vi "Remove Headers from XML.vi"(8 "error in (no error)":errorcluster, 10 "XML (with headers)":string) -> (0 "error out":errorcluster, 2 "XML (without headers)":string)   [LabVIEW 2013]
panel:
  # "Copyright © 2007 James Kring, Inc. All rights reserved.\n\nAuthor: Jim Kring <jim.kring@jameskring.com>\n\nThis library is provided \"AS IS\" , WITHOUT WARRANTIES OR \nCONDITIONS OF ANY KIND, either express or implied.\n\nJames Kring, Inc. -- http://www.jameskring.com"
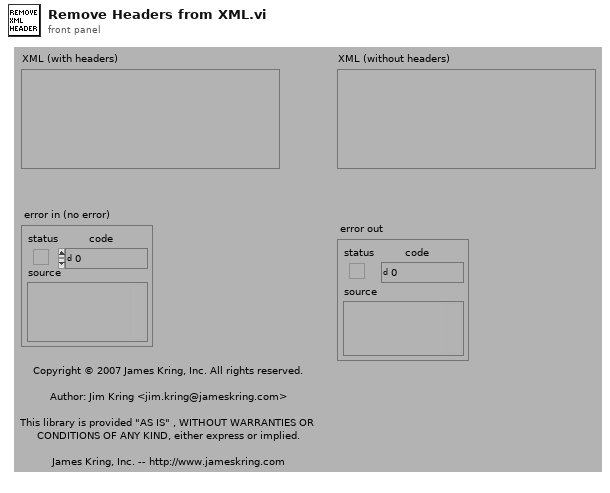
[diagram p1: front panel]
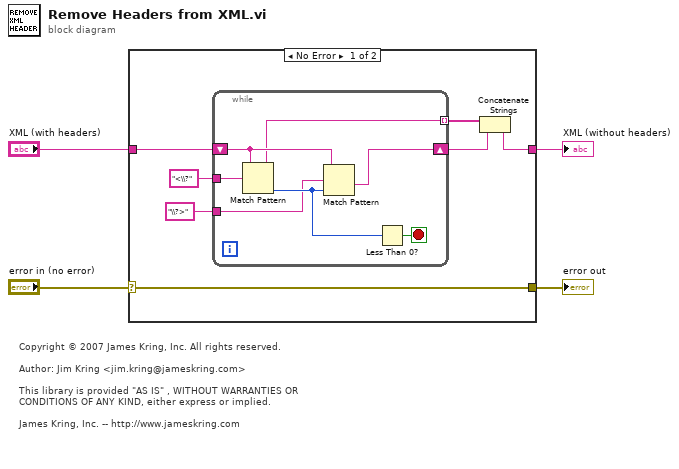
[diagram p0: block diagram]
diagram:
  # "Copyright © 2007 James Kring, Inc. All rights reserved.\n\nAuthor: Jim Kring <jim.kring@jameskring.com>\n\nThis library is provided \"AS IS\" , WITHOUT WARRANTIES OR \nCONDITIONS OF ANY KIND, either express or implied.\n\nJames Kring, Inc. -- http://www.jameskring.com"
  n1 = case shown="No Error" "error in (no error)" {
    selector: "error in (no error)" -> [w5 w19]
    tunnel: [w9 _] -> w4
    tunnel: "XML (with headers)" -> [w8 _]
    tunnel: [w5 w19] -> w2
    frame No Error {
      n2 = while {
        tunnel: "<\\?" ("regular expression") -> [w18]
        shift-right: [w14] -> w10
        shift-left: w8 -> [w15]
        tunnel: "\\?>" ("regular expression") -> [w13]
        tunnel: [w12] -> w6 mode=indexing
        stop <- w17 stop-if-true
        n3 = Match Pattern(string=w15, regular expression=w18) -> (before substring=w12:string, offset past match=w16:i32)  [unwired: 1 in, 2 out]
        n4 = Match Pattern(string=w15, regular expression=w13, offset (0)=w16) -> (after substring=w14:string)  [unwired: 3 out]
        n5 = Less Than 0?(x=w16) -> (x < 0?=w17:bool)
      }
      n6 = Concatenate Strings(w6, w10) -> (w9:string)
    }
    frame Error {
    }
  }
  "XML (without headers)" <- w4
  "error out" <- w2
